vi "slave_vi.vi"() -> (2 "ref to control on another VI":refnum<vi>)   [LabVIEW 2021]
panel:
  out "control on another VI":bool
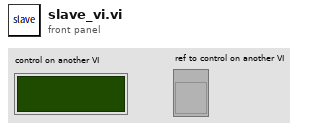
[diagram p1: front panel]
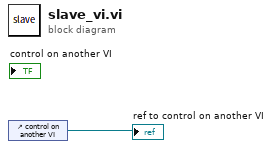
[diagram p0: block diagram]
diagram:
  n1 = control-ref of="control on another VI"() -> (→"ref to control on another VI":refnum<vi>)
